vi "appendArray.vi"(1 "input array":u8[](array[numeric]), 2 "element":u8=1) -> (0 "output":u8[](array[numeric]))   [LabVIEW 2013]
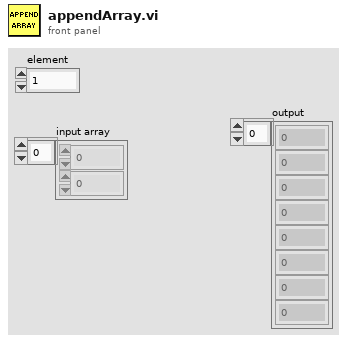
[diagram p1: front panel]
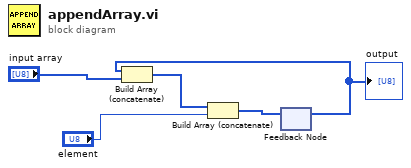
[diagram p0: block diagram]
diagram:
  n1 = feedback #1() -> (w1:u8[])  [unwired: 1 in]
  "output" <- w1
  n2 = Build Array (concatenate)(w1, "input array") -> (w5:u8[])
  n3 = Build Array (concatenate)(w5, "element") -> (w2:u8[])
  n4 = feedback-in #1(w2) -> ()
